vi "Get Mentions New.vi"(8 "error in":errorcluster, 9 "Mentions to Read (10)":i32=10 min=0 max=200 step=1, 11 "Twitter Handle In":T2={"OAuth Credentials"={"Consumer Key"="", "Signature Method"=enum."HMAC-SHA1", "Token"="", "Version"="", "Token Secret"="", "Consumer Secret"=""}, "since ID"="", "max ID"="", "Screen Name"=""}) -> (0 "error out":errorcluster, 1 "Actual Num of Mentions Read":i32, 2 "New Mentions Read":T1[](array[typedef]), 3 "Twitter Handle Out":T2={"OAuth Credentials"={"Consumer Key"="", "Signature Method"=enum."HMAC-SHA1", "Token"="", "Version"="", "Token Secret"="", "Consumer Secret"=""}, "since ID"="", "max ID"="", "Screen Name"=""}, 5 "Time Stamp of Newest Mention":timestamp)   [LabVIEW 2011, in "i3-twitter.lvlib"]
doc: "Get authenticating user's new mentions."
uses:
  i3-twitter.lvlib
  Controls/Twitter Handle.ctl
  i3-oauth/Controls/OAuth Credentials.ctl
  i3-oauth/Controls/Signature Method.ctl
  Controls/Tweet.ctl
  i3-oauth/Controls/HTTP Method.ctl
  i3-json/JSON Parsing/Get Array Value at Index Files/Get Array Value at Index - Object.vi
  i3-json/JSON Parsing/Get Object Parameter Files/Get Object Parameter - String.vi
  i3-json/JSON Parsing/Get Object Parameter Files/Get Object Parameter - Object.vi
  i3-oauth/i3-oauth.lvlib
  <vilib>/httpClient/LabVIEWHTTPClient.lvlib
  i3-json/i3-json.lvlib
panel:
  out "headers":string
  out "body":string
  out "Full URL":string
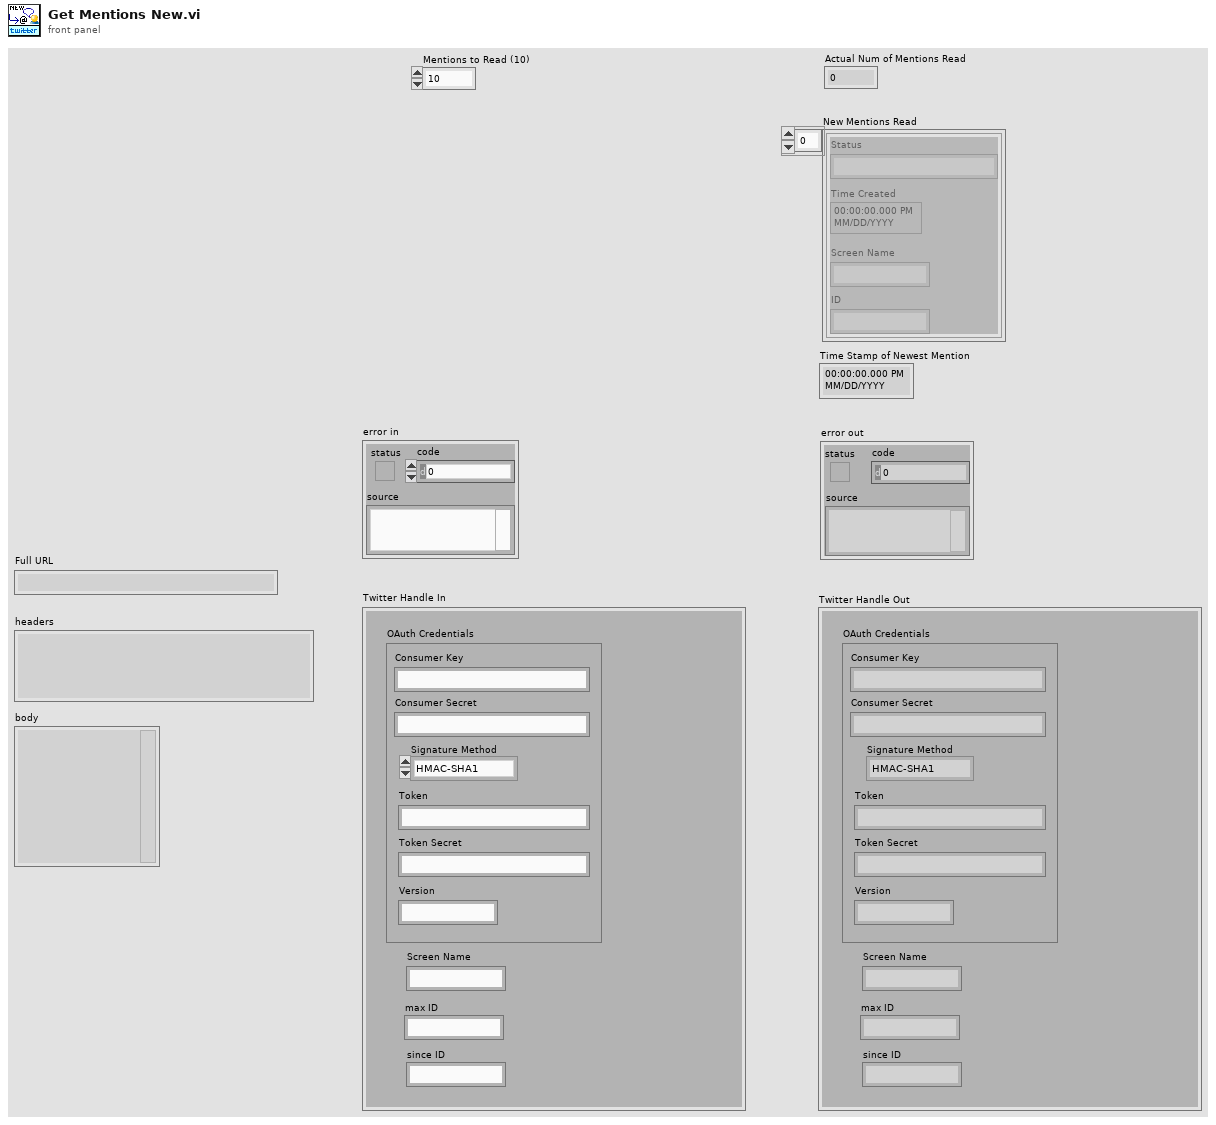
[diagram p1: front panel]
types:
  T1 = typedef "i3-twitter.lvlib/Tweet.ctl" = cluster{"Status":string, "Time Created":timestamp, "Screen Name":string, "ID":string}
  T2 = typedef "i3-twitter.lvlib/Twitter Handle.ctl" = cluster{"OAuth Credentials":T3, "since ID":string, "max ID":string, "Screen Name":string}
  T3 = typedef "i3-oauth.lvlib/OAuth Credentials.ctl" = cluster{"Consumer Key":string, "Signature Method":T4, "Token":string, "Version":string, "Token Secret":string, "Consumer Secret":string}
  T4 = typedef "i3-oauth.lvlib/Signature Method.ctl" = enum16{"HMAC-MD5", "HMAC-SHA1", "HMAC-SHA224", "HMAC-SHA256", "HMAC-SHA384", "HMAC-SHA512"}
  T5 = typedef "i3-oauth.lvlib/HTTP Method.ctl" = enum16{"GET", "POST", "PUT", "DELETE"}
  T6 = typedef "i3-oauth.lvlib/key-value-pairs.ctl" = cluster{"key":string, "value":string}
  T7 = typedef "LabVIEWHTTPClient.lvlib/ClientHandle.ctl" = refnum<k1>
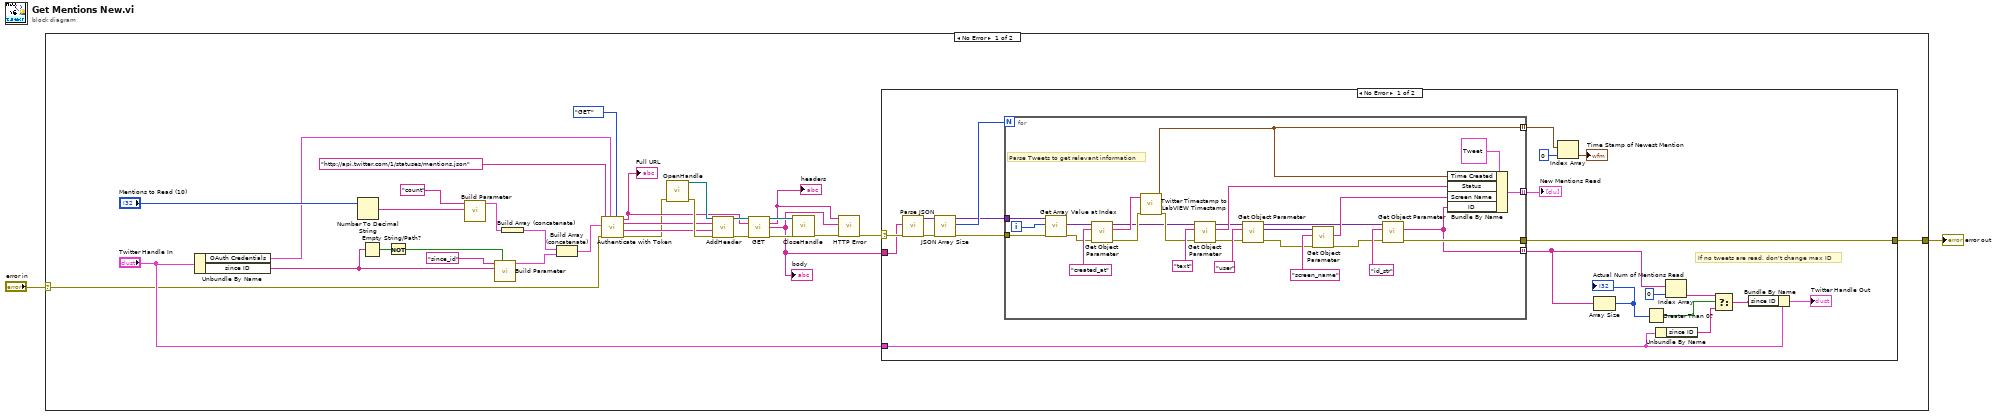
[diagram p0: block diagram]
diagram:
  n1 = case shown="No Error" "error in" {
    selector: "error in" -> [w3 w83]
    tunnel: [w6 w83] -> w2
    frame No Error {
      n2 = Unbundle By Name("Twitter Handle In") -> ("OAuth Credentials"=w16:T3, "since ID"=w4:string)
      n3 = Number To Decimal String(number="Mentions to Read (10)") -> (decimal integer string=w20:string)  [unwired: 1 in]
      n4 = Empty String/Path?(string/path=w4) -> (empty?=w14:bool)
      n5 = Not(x=w14) -> (.not. x?=w11:bool)
      n6 = call "Build Parameter.vi"("Value"=w20, "Key"="count") -> ("Parameter Array"=w19:T6[])  [unwired: 9 in]
      n7 = call "Build Parameter.vi"("Return Parameter? (T)"=w11, "Value"=w4, "Key"="since_id") -> ("Parameter Array"=w13:T6[])  [unwired: 8 in]
      n8 = Build Array (concatenate)(w19) -> (w18:T6[])
      n9 = Build Array (concatenate)(w18, w13) -> (w17:T6[])
      n10 = call "Authenticate with Token.vi"("HTTP Method"=HTTP_Method."GET", "OAuth Credentials"=w16, "error in (no error)"=w3, "URL Parameters"=w17, "Base URL"="http://api.twitter.com/1/statuses/mentions.json") -> ("error out"=w15:errorcluster, "Header Value"=w25:string, "Header Parameter"=w26:string, "Full URL"=w23:string)  [unwired: 2 in, 1 out]
      "Full URL" <- w23
      n11 = call <vilib>:"OpenHandle.vi"("error in (no error)"=w15) -> ("client handle out"=w32:T7, "error out"=w31:errorcluster)  [unwired: 13 in]
      n12 = call <vilib>:"AddHeader.vi"("client handle"=w32, "header"=w26, "value"=w25, "error in (no error)"=w31) -> ("client handle out"=w30:T7, "error out"=w29:errorcluster)  [unwired: 10 in]
      n13 = call <vilib>:"GET.vi"("client handle"=w30, "url"=w23, "error in (no error)"=w29) -> ("client handle out"=w28:T7, "headers"=w10:string, "body"=w5:string, "error out"=w27:errorcluster)  [unwired: 9 in]
      "body" <- w5
      "headers" <- w10
      n14 = call <vilib>:"CloseHandle.vi"("client handle"=w28, "error in (no error)"=w27) -> ("error out"=w9:errorcluster)  [unwired: 13 in]
      n15 = call "HTTP Error.vi"("error in (no error)"=w9, "Body"=w5, "Header"=w10) -> ("error out"=w7:errorcluster)  [unwired: 6 in, 2 out]
      n16 = case shown="No Error" w7 {
        selector: w7 -> [w43 w82]
        tunnel: "Twitter Handle In" -> [w34 _]
        tunnel: [w42 w82] -> w6
        tunnel: w5 -> [w41 _]
        frame No Error {
          # "If no tweets are read, don't change max ID"
          n17 = call "Parse JSON.vi"("error in (no error)"=w43, "JSON String"=w41) -> ("error out"=w51:errorcluster, "JSON Tree"=w53:variant)  [unwired: 6 in, 2 out]
          n18 = call "JSON Array Size.vi"("error in (no error)"=w51, "JSON Tree In (JSON Array)"=w53) -> ("error out"=w50:errorcluster, "Array Size"=w54:i32, "JSON Tree Passthrough (JSON Array)"=w44:variant)  [unwired: 7 in]
          n19 = for {
            N: w54 -> [_]
            tunnel: [w69] -> w52 mode=indexing
            tunnel: w50 -> [w65]
            tunnel: [w71] -> w49 mode=indexing
            tunnel: [w70] -> w42
            tunnel: w44 -> [w64]
            tunnel: [w63] -> w40 mode=indexing
            i -> [w75]
            # "Parse Tweets to get relevant information"
            n20 = call-poly "Get Array Value at Index.vi"("error in (no error)"=w65, "Index"=w75, "JSON Tree In (JSON Array)"=w64) -> ("error out"=w73:errorcluster, "JSON Object"=w61:variant)  [unwired: 5 in, 2 out]
            n21 = call-poly "Get Object Parameter.vi"("error in (no error)"=w73, "Parameter Name"="created_at", "JSON Tree In (JSON Object)"=w61) -> ("error out"=w60:errorcluster, "String Value"=w59:string, "JSON Tree Out Passthrough"=w57:variant)  [unwired: 5 in, 1 out]
            n22 = call "Twitter Timestamp to LabVIEW Timestamp.vi"("error in"=w60, "Twitter Time Stamp"=w59) -> ("error out"=w68:errorcluster, "LabVIEW Time Stamp"=w63:timestamp)  [unwired: 6 in]
            n23 = call-poly "Get Object Parameter.vi"("error in (no error)"=w68, "Parameter Name"="text", "JSON Tree In (JSON Object)"=w57) -> ("error out"=w58:errorcluster, "String Value"=w66:string, "JSON Tree Out Passthrough"=w56:variant)  [unwired: 5 in, 1 out]
            n24 = call-poly "Get Object Parameter.vi"("error in (no error)"=w58, "Parameter Name"="user", "JSON Tree In (JSON Object)"=w56) -> ("error out"=w72:errorcluster, "JSON Object"=w62:variant, "JSON Tree Out Passthrough"=w55:variant)  [unwired: 5 in, 1 out]
            n25 = call-poly "Get Object Parameter.vi"("error in (no error)"=w72, "Parameter Name"="screen_name", "JSON Tree In (JSON Object)"=w62) -> ("error out"=w67:errorcluster, "String Value"=w78:string)  [unwired: 5 in, 2 out]
            n26 = call-poly "Get Object Parameter.vi"("error in (no error)"=w67, "Parameter Name"="id_str", "JSON Tree In (JSON Object)"=w55) -> ("error out"=w70:errorcluster, "String Value"=w69:string)  [unwired: 5 in, 2 out]
            n27 = Bundle By Name(cluster=T1 {"Status"="", "Time Created"=timestamp(0 s since 1904-01-01), "Screen Name"="", "ID"=""}, "Time Created"=w63, "Status"=w66, "Screen Name"=w78, "ID"=w69) -> (w71:T1)
          }
          "New Mentions Read" <- w49
          n28 = Index Array(array=w40, index=0) -> (element=→"Time Stamp of Newest Mention":timestamp)
          n29 = Array Size(array=w52) -> (size(s)=w47:i32)
          "Actual Num of Mentions Read" <- w47
          n30 = Greater Than 0?(x=w47) -> (x > 0?=w48:bool)
          n31 = Unbundle By Name(w34) -> ("since ID"=w35:string)
          n32 = Index Array(array=w52, index=0) -> (element=w46:string)
          n33 = Select(t=w46, s=w48, f=w35) -> (s? t:f=w45:string)
          n34 = Bundle By Name(cluster=w34, "since ID"=w45) -> (→"Twitter Handle Out":T2)
        }
        frame Error {
        }
      }
    }
    frame Error {
    }
  }
  "error out" <- w2
